vi "Values String Changed.vi"(8 "error in (no error)":errorcluster, 11 "Application Data in":T1={"Item Tree Control"=refnum, "Top-Level VI"=refnum, "menu reference"=refnum, "queue"=refnum, "Stop Pointer"=refnum, "Buffer Variant"=variant, "server ID"=refnum, "framework tag"="", "Values"=refnum, "Hex"=refnum, "ASCII"=refnum, "lines visible"=0, "values padding"=0, "current buffer data"={"decimation"=0, "avg bandwidth"=0.0, "channels"=[], "byte order"=enum."little-endian", "buffer descriptor"={"buffer type"=enum."Engine", "plugin id"=0, "group id"=0, "transfer id"=0, "offset"=0, "length"=0}, "values channels"={"index"=0, "count"=0, "engine offset"=0}, "select start offset"=18446744073709551615, "select end offset"=0, "channel index"=-1}, "Framework Configuration"=refnum} {"current buffer data"."channels"."configuration"."string offset" format="%d bytes"; "current buffer data"."avg bandwidth" format="%.0g bytes"}) -> (0 "error out":errorcluster, 3 "Application Data out":T1={"Item Tree Control"=refnum, "Top-Level VI"=refnum, "menu reference"=refnum, "queue"=refnum, "Stop Pointer"=refnum, "Buffer Variant"=variant, "server ID"=refnum, "framework tag"="", "Values"=refnum, "Hex"=refnum, "ASCII"=refnum, "lines visible"=0, "values padding"=0, "current buffer data"={"decimation"=0, "avg bandwidth"=0.0, "channels"=[], "byte order"=enum."little-endian", "buffer descriptor"={"buffer type"=enum."Engine", "plugin id"=0, "group id"=0, "transfer id"=0, "offset"=0, "length"=0}, "values channels"={"index"=0, "count"=0, "engine offset"=0}, "select start offset"=18446744073709551615, "select end offset"=0, "channel index"=-1}, "Framework Configuration"=refnum} {"current buffer data"."channels"."configuration"."string offset" format="%d bytes"; "current buffer data"."avg bandwidth" format="%.0g bytes"})   [LabVIEW 2017, in "DSF Core.lvlib"]
uses:
  DSF Core.lvlib
  Application Data.ctl
  <vilib>/NI/Memory Manager/Classes/Pointer/Pointer.lvclass
  Classes/Configuration/Framework/Framework Configuration.lvclass
  Buffer Reader/Queue Data.ctl
  Buffer Reader/Buffer Data.ctl
  Classes/Configuration/Base/Transfer/Channel Configuration.ctl
  Typedefs/Core Channel Configuration.ctl
  Typedefs/DSF Data Type.ctl
  Typedefs/DSF Settings Info.ctl
  Typedefs/DSF Byte Order.ctl
  Classes/Thread/Data Server/DSF Buffer Subset Descriptor.ctl
  Typedefs/DSF Buffer Type.ctl
  Values Channels.ctl
  Classes/Framework/Framework.lvclass
  Classes/Configuration/Base/Channel/Channel Configuration.lvclass
  Classes/Configuration/Base/Transfer/Transfer Configuration.lvclass
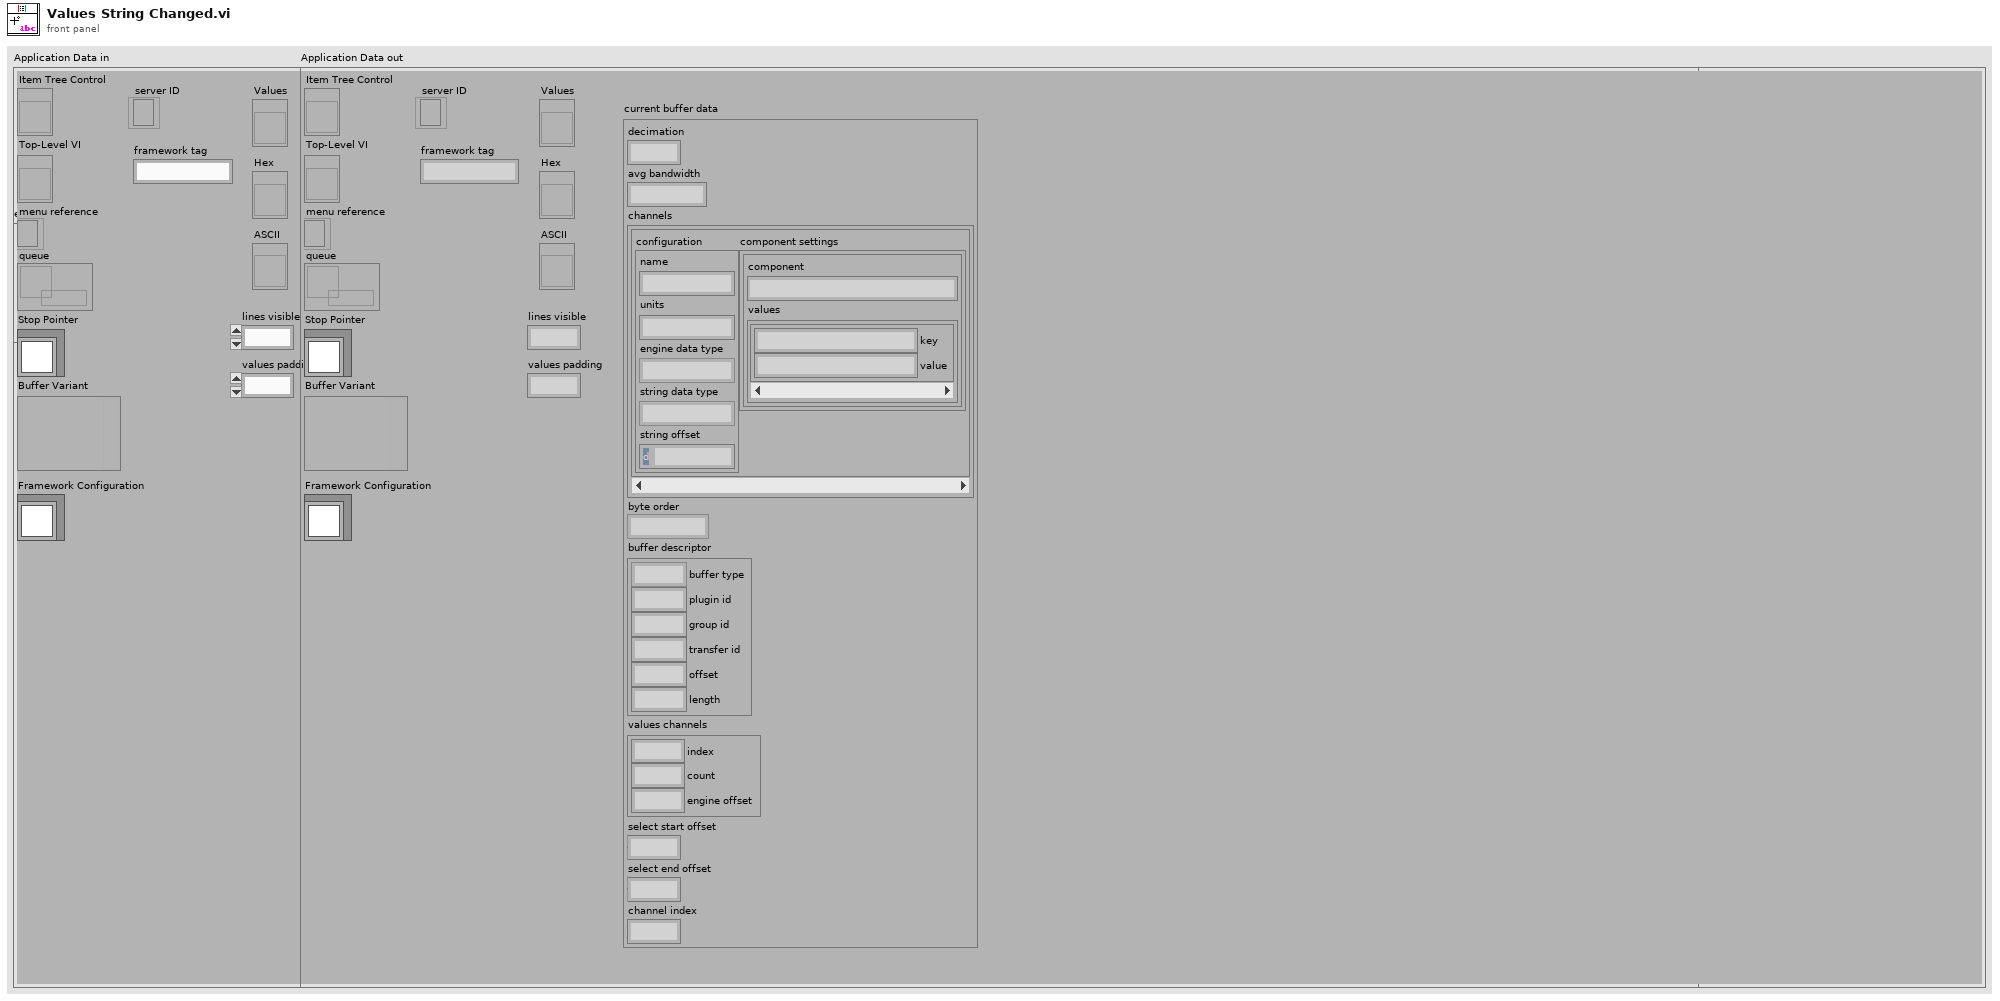
[diagram p1: front panel]
types:
  T1 = typedef "DSF Core.lvlib/Application Data.ctl" = cluster{"Item Tree Control":refnum<vi>, "Top-Level VI":refnum<vi>, "menu reference":refnum<k9>, "queue":refnum<queue>, "Stop Pointer":refnum<class "Pointer.lvclass">, "Buffer Variant":variant, "server ID":refnum<k5>, "framework tag":string, "Values":refnum<vi>, "Hex":refnum<vi>, "ASCII":refnum<vi>, "lines visible":i32, "values padding":i32, "current buffer data":T2, "Framework Configuration":refnum<class "Framework Configuration.lvclass">}
  T2 = typedef "DSF Core.lvlib/Buffer Data.ctl" = cluster{"decimation":u64, "avg bandwidth":dbl, "channels":T3[], "byte order":T7, "buffer descriptor":T8, "values channels":T10, "select start offset":u64, "select end offset":u64, "channel index":i32}
  T3 = typedef "DSF Core.lvlib/Transfer Configuration.lvclass/Channel Configuration.ctl" = cluster{"configuration":T4, "component settings":T6[]}
  T4 = typedef "DSF Core.lvlib/Channel Configuration.lvclass/Core Channel Configuration.ctl" = cluster{"name":string, "units":string, "engine data type":T5, "string data type":T5, "string offset":u64}
  T5 = typedef "DSF Core.lvlib/DSF Data Type.ctl" = enum8{"Bool", "SGL", "DBL", "I8", "I16", "I32", "I64", "U8", "U16", "U32", "U64"}
  T6 = typedef "DSF Core.lvlib/DSF Settings Info.ctl" = cluster{"component":string, "values":cluster{"key":string, "value":string}[]}
  T7 = typedef "DSF Core.lvlib/DSF Byte Order.ctl" = enum8{"big-endian", "little-endian"}
  T8 = typedef "DSF Core.lvlib/DSF Buffer Subset Descriptor.ctl" = cluster{"buffer type":T9, "plugin id":i32, "group id":i32, "transfer id":i32, "offset":u64, "length":i64}
  T9 = typedef "DSF Core.lvlib/DSF Buffer Type.ctl" = enum16{"Engine", "String"}
  T10 = typedef "DSF Core.lvlib/Values Channels.ctl" = cluster{"index":i32, "count":i32, "engine offset":u64}
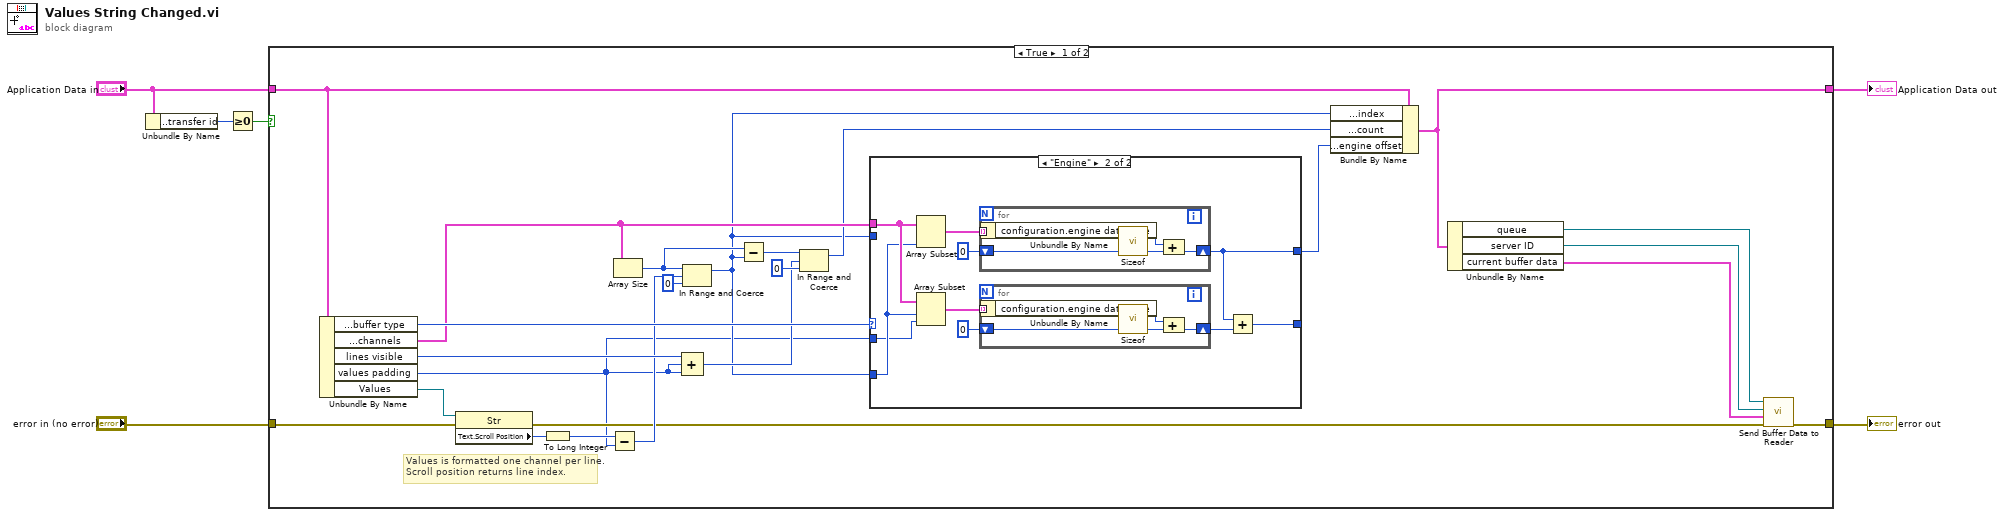
[diagram p0: block diagram]
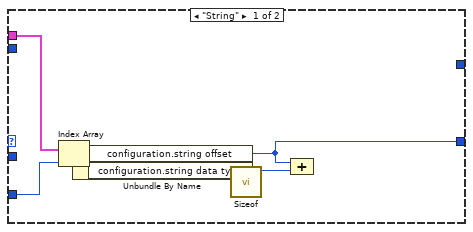
[diagram p2: hidden frame]
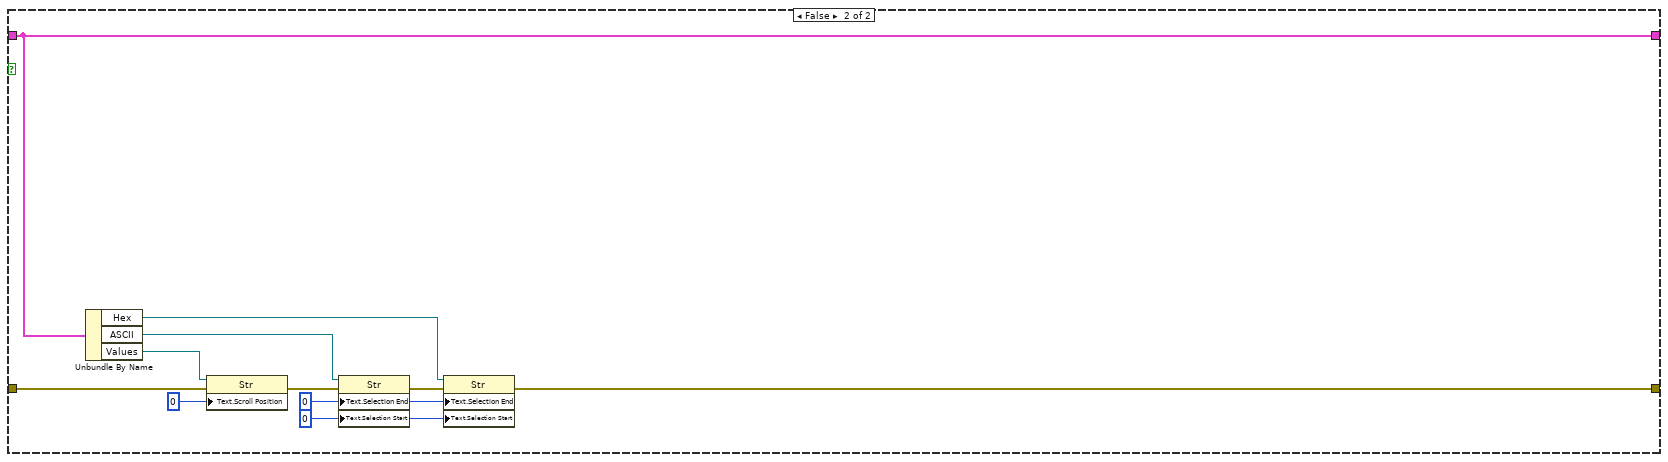
[diagram p3: hidden frame]
diagram:
  n1 = Unbundle By Name("Application Data in") -> ("current buffer data.buffer descriptor.transfer id"=w1:i32)
  n2 = Greater Or Equal To 0?(x=w1) -> (x >= 0?=w2:bool)
  n3 = case shown="True" w2 {
    tunnel: "error in (no error)" -> [w30 w66]
    tunnel: [w22 w63] -> w4
    tunnel: "Application Data in" -> [w25 w65]
    tunnel: [w18 w65] -> w5
    frame True {
      # "Values is formatted one channel per line. Scroll position returns line index."
      n4 = Unbundle By Name(w25) -> ("current buffer data.buffer descriptor.buffer type"=w24:T9, "current buffer data.channels"=w23:T3[], "lines visible"=w16:i32, "values padding"=w7:i32, "Values"=w26:refnum<vi>)
      n5 = property class="Str"(reference=w26, error in=w30) -> (error out=w8:errorcluster, "Text.Scroll Position"=w28:u32)  [unwired: 1 out]
      n6 = To Long Integer(number=w28) -> (32bit integer=w27:i32)
      n7 = Subtract(x=w27, y=w7) -> (x-y=w15:i32)
      n8 = Array Size(array=w23) -> (size(s)=w14:i32)
      n9 = Compound Arithmetic op=ADD(w16, w7, w7) -> (w10:i32)
      n10 = In Range and Coerce(upper limit=w14, x=w15, lower limit=0) -> (coerced(x)=w9:i32)  [unwired: 1 out]
      n11 = Subtract(x=w14, y=w9) -> (x-y=w12:i32)
      n12 = In Range and Coerce(upper limit=w12, x=w10, lower limit=0) -> (coerced(x)=w11:i32)  [unwired: 1 out]
      n13 = case shown="\"Engine\"" w24 {
        tunnel: w23 -> [w34 w43]
        tunnel: w9 -> [_ _]
        tunnel: w9 -> [w33 w41]
        tunnel: [w31 w37] -> _
        tunnel: [_ w38] -> w17
        tunnel: w7 -> [_ w40]
        frame "String" {
          n14 = Index Array(array=w34, index=w33) -> (element=w32:T3)
          n15 = Unbundle By Name(w32) -> ("configuration.string offset"=w31:u64, "configuration.string data type"=w36:T5)
          n16 = call "Sizeof.vi"("data type"=w36) -> ("size in bytes"=w35:u64)  [unwired: 9 in, 1 out]
          n17 = Compound Arithmetic op=ADD(w31, w35) -> ()  [unwired: 1 out]
        }
        frame "Engine" {
          n18 = Array Subset(array=w43, length=w41) -> (w45:T3[])  [unwired: 1 in]
          n19 = Array Subset(array=w43, index=w41, length=w40) -> (w42:T3[])
          n20 = for {
            tunnel: w45 -> [w56] mode=indexing
            shift-right: [w53] -> w38
            shift-left: u64 0 ("value") -> [w54]
            n21 = Unbundle By Name(w56) -> ("configuration.engine data type"=w55:T5)
            n22 = call "Sizeof.vi"("data type"=w55) -> ("size in bytes"=w52:u64)  [unwired: 9 in, 1 out]
            n23 = Compound Arithmetic op=ADD(w52, w54) -> (w53:u64)
          }
          n24 = for {
            tunnel: w42 -> [w51] mode=indexing
            shift-right: [w48] -> w39
            shift-left: u64 0 ("value") -> [w49]
            n25 = Unbundle By Name(w51) -> ("configuration.engine data type"=w50:T5)
            n26 = call "Sizeof.vi"("data type"=w50) -> ("size in bytes"=w47:u64)  [unwired: 9 in, 1 out]
            n27 = Compound Arithmetic op=ADD(w47, w49) -> (w48:u64)
          }
          n28 = Add(x=w38, y=w39) -> (x+y=w37:u64)
        }
      }
      n29 = Bundle By Name(cluster=w25, "current buffer data.values channels.index"=w9, "current buffer data.values channels.count"=w11, "current buffer data.values channels.engine offset"=w17) -> (w18:T1)
      n30 = Unbundle By Name(w18) -> ("queue"=w19:refnum<queue>, "server ID"=w20:refnum<k5>, "current buffer data"=w21:T2)
      n31 = call "Send Buffer Data to Reader.vi"("error in (no error)"=w8, "Buffer data"=w21, "server ID"=w20, "queue"=w19) -> ("error out"=w22:errorcluster)  [unwired: 7 in]
    }
    frame False {
      w58 = u32 0 ("Text.Selection:Start")
      w57 = u32 0 ("Text.Selection:End")
      n32 = Unbundle By Name(w65) -> ("Hex"=w59:refnum<vi>, "ASCII"=w60:refnum<vi>, "Values"=w62:refnum<vi>)
      n33 = property class="Str"(reference=w62, error in=w66, "Text.Scroll Position"=u32 0) -> (error out=w67:errorcluster)  [unwired: 1 out]
      n34 = property class="Str"(reference=w60, error in=w67, "Text.Selection End"=w57, "Text.Selection Start"=w58) -> (error out=w64:errorcluster)  [unwired: 1 out]
      n35 = property class="Str"(reference=w59, error in=w64, "Text.Selection End"=w57, "Text.Selection Start"=w58) -> (error out=w63:errorcluster)  [unwired: 1 out]
    }
  }
  "error out" <- w4
  "Application Data out" <- w5
